vi "Run_Device.vi"(8 "error in (no error)":errorcluster, 10 "Message_command":T2, 11 "Command Queue":T3) -> (0 "error out":errorcluster, 2 "dup Message_command":T2, 3 "dup Command Queue":T3)   [LabVIEW 2020]
uses:
  Command_Queue.ctl
  Command_Message.ctl
  Device_List.ctl
panel:
  in  "Device":T1
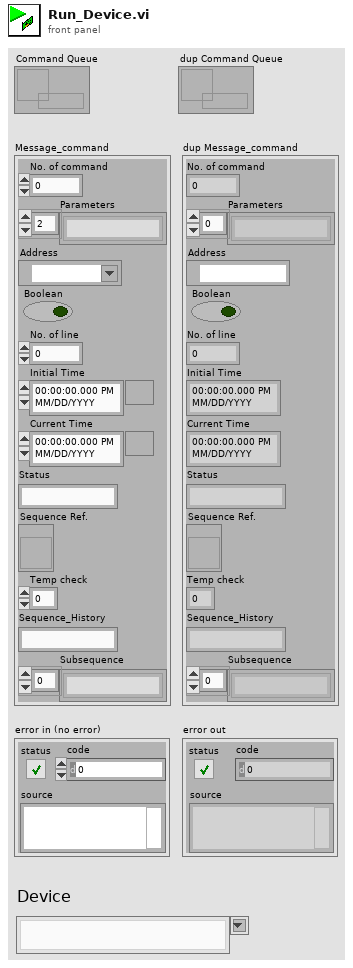
[diagram p1: front panel]
types:
  T1 = typedef "Device_List.ctl" = string
  T2 = typedef "Command_Message.ctl" = cluster{"No. of command":i32, "Parameters":string[], "Address":refnum<visa-resource-name>, "Boolean":bool, "No. of line":i32, "Initial Time":timestamp, "Current Time":timestamp, "Status":string, "Sequence Ref.":refnum<vi>, "Temp check":i32, "Sequence_History":string, "Subsequence":string[]}
  T3 = typedef "Command_Queue.ctl" = refnum<queue>
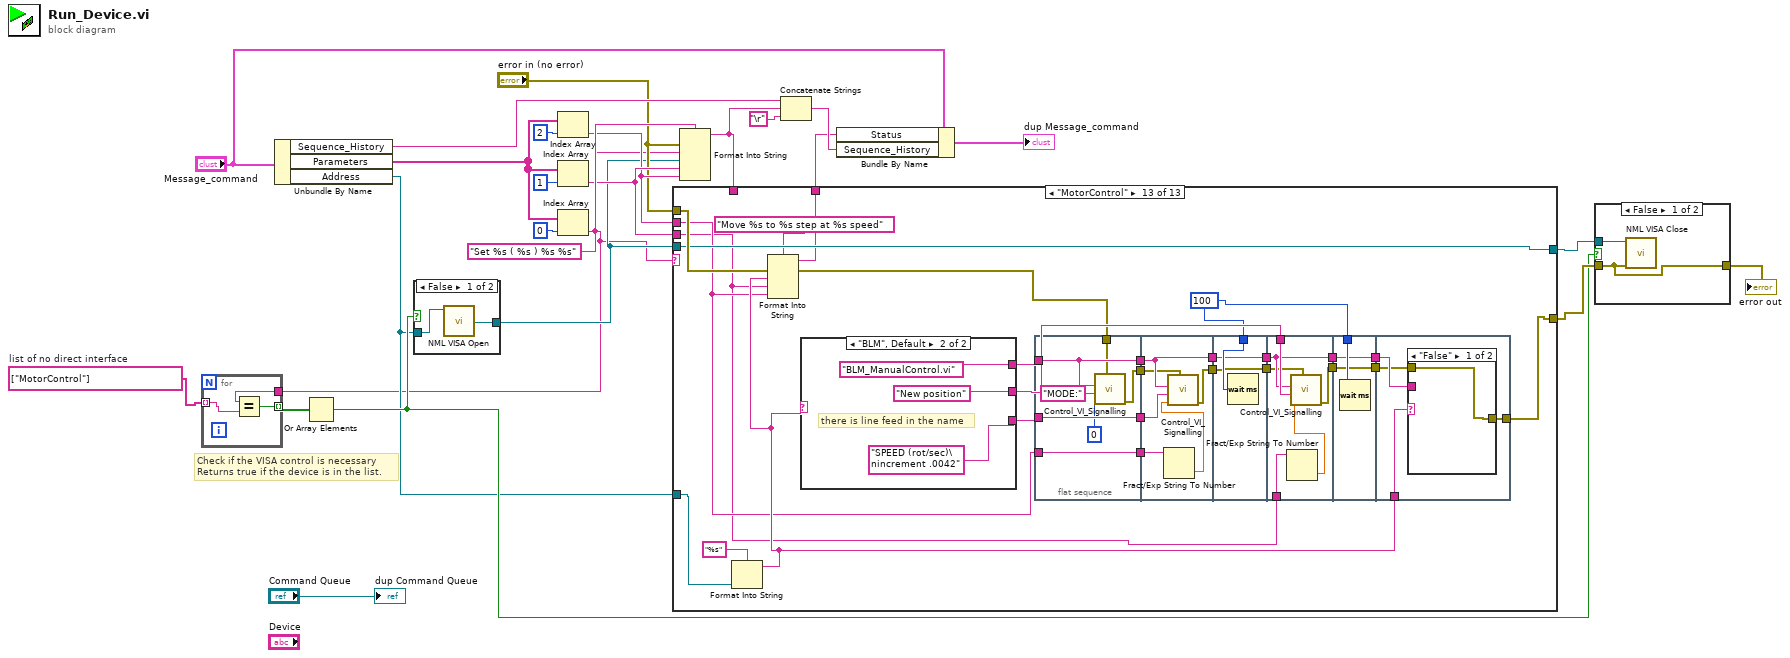
[diagram p0: block diagram]
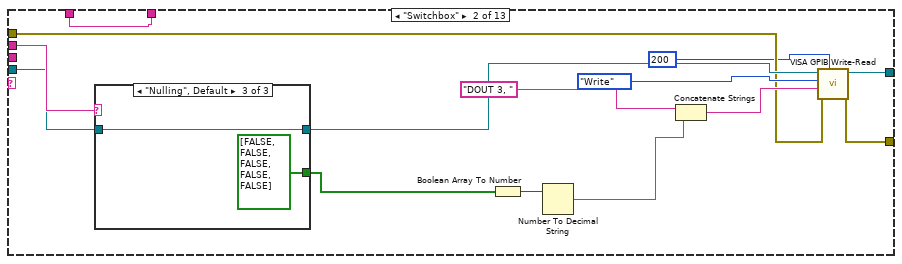
[diagram p5: hidden frame]
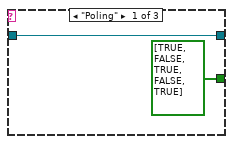
[diagram p6: hidden frame]
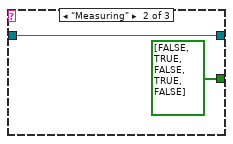
[diagram p7: hidden frame]
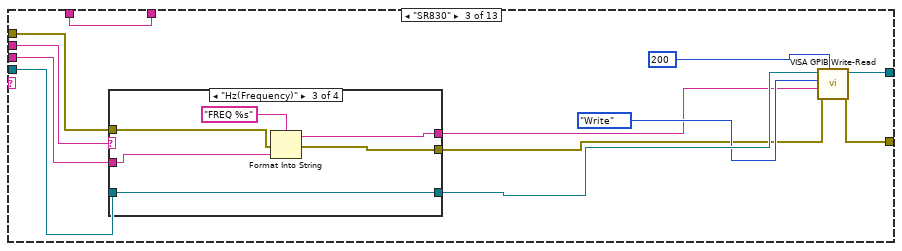
[diagram p8: hidden frame]
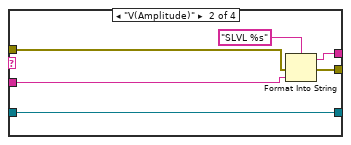
[diagram p10: hidden frame]
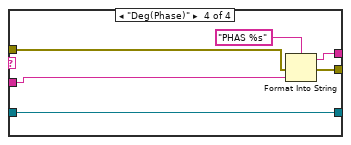
[diagram p11: hidden frame]
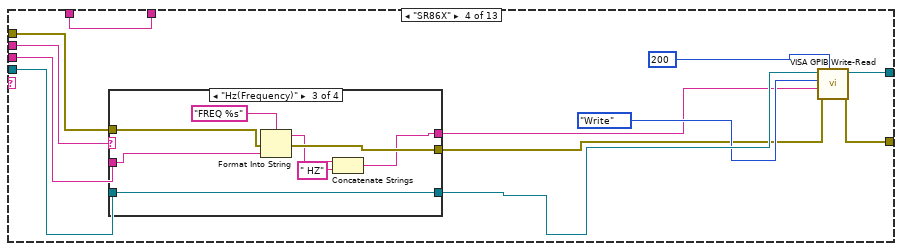
[diagram p12: hidden frame]
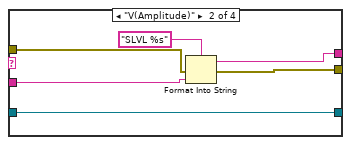
[diagram p14: hidden frame]
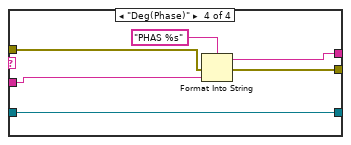
[diagram p15: hidden frame]
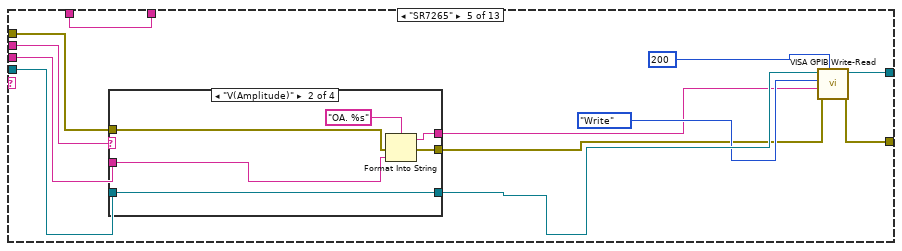
[diagram p16: hidden frame]
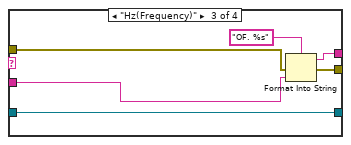
[diagram p18: hidden frame]
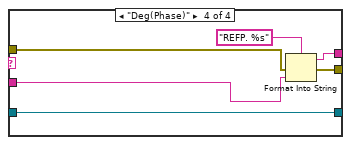
[diagram p19: hidden frame]
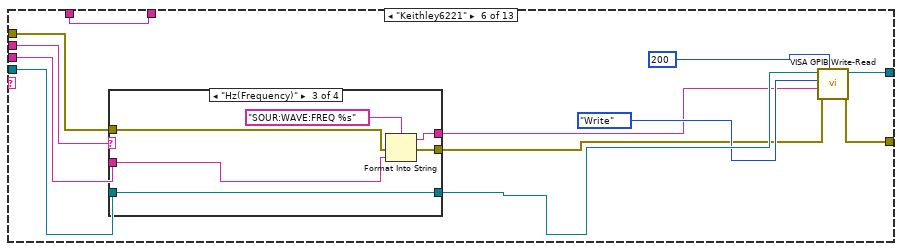
[diagram p20: hidden frame]
diagram:
  w7 = string[] ["MotorControl"]  # list of no direct interface
  # "Check if the VISA control is necessary\nReturns true if the device is in the list."
  n1 = Unbundle By Name("Message_command") -> ("Sequence_History"=w17:string, "Parameters"=w12:string[], "Address"=w4:refnum<visa-resource-name>)
  n2 = Index Array(array=w12, index=2) -> (element=w19:string)
  n3 = Index Array(array=w12, index=1) -> (element=w20:string)
  n4 = Index Array(array=w12, index=0) -> (element=w1:string)
  n5 = for {
    tunnel: w7 -> [w27] mode=indexing
    tunnel: w1 -> [w28]
    tunnel: [w26] -> w6 mode=indexing
    n6 = Equal?(x=w28, y=w27) -> (x = y?=w26:bool)
  }
  n7 = Or Array Elements(Boolean array=w6) -> (logical OR=w5:bool)
  n8 = case shown="False" w5 {
    tunnel: w4 -> [w30 w31]
    tunnel: [w29 w31] -> w11
    frame False {
      n9 = call "NML VISA Open.vi"("VISA resource name"=w30) -> ("VISA resource name out"=w29:refnum<visa-resource-name>)  [unwired: 9 in, 1 out]
    }
    frame True {
    }
  }
  n10 = Format Into String(format string="Set %s ( %s ) %s %s", error in="error in (no error)", w1, w11, w20, w19) -> (resulting string=w3:string)  [unwired: 1 in, 1 out]
  n11 = case shown="\"MotorControl\"" w1 {
    tunnel: w19 -> [_ w48 w66 w99 w134 w167 w202 w224 w315 w377 w440 w479 w521]
    tunnel: w20 -> [_ _ w64 w97 w132 w165 w200 w222 w313 w375 w436 w475 w520]
    tunnel: w11 -> [w33 w47 w63 w96 w131 w164 w199 w221 w312 w374 w437 w476 w524]
    tunnel: "error in (no error)" -> [w34 w39 w65 w98 w133 w166 w201 w223 w314 w376 w439 w478 w525]
    tunnel: [w34 w38 w58 w91 w126 w159 w194 w216 w307 w369 w438 w477 w512] -> w9
    tunnel: [w33 w36 w56 w89 w124 w157 w192 w214 w305 w367 w435 w474 w524] -> w10
    tunnel: w4 -> [_ _ _ _ _ _ _ _ _ _ _ _ w526]
    tunnel: w3 -> [w32 w35 w55 w88 w123 w156 w191 w213 w304 w366 w434 w473 _]
    tunnel: [w32 w35 w55 w88 w123 w156 w191 w213 w304 w366 w434 w473 w519] -> w2
    frame "False", Default {
    }
    frame "Switchbox" {
      n12 = case shown="\"Nulling\", Default" w48 {
        tunnel: w47 -> [w50 w51 w53]
        tunnel: [w50 w51 w53] -> w46
        tunnel: [bool[] [TRUE, FALSE, TRUE, FALSE, TRUE] bool[] [FALSE, TRUE, FALSE, TRUE, FALSE] bool[] [FALSE, FALSE, FALSE, FALSE, FALSE]] -> w41
        frame "Poling" {
        }
        frame "Measuring" {
        }
        frame "Nulling", Default {
        }
      }
      n13 = Boolean Array To Number(Boolean array=w41) -> (number=w42:u32)
      n14 = Number To Decimal String(number=w42) -> (decimal integer string=w44:string)  [unwired: 1 in]
      n15 = Concatenate Strings("DOUT 3, " ("string"), w44) -> (w40:string)
      n16 = call "VISA GPIB Write-Read.vi"("Wait (ms)"=u32 200 ("wait (mS)"), "error in (no error)"=w39, "Command"=w40, "Action"=enum16{"Write", "Read", "Write & Read"}."Write", "VISA resource name"=w46) -> ("error out"=w38:errorcluster, "dup VISA Session"=w36:refnum<visa-resource-name>)  [unwired: 3 in, 2 out]
    }
    frame "SR830" {
      n17 = case shown="\"Hz(Frequency)\"" w66 {
        selector: w66 -> [w67 _ _ _]
        tunnel: w65 -> [w69 w74 w80 w86]
        tunnel: [w69 w72 w78 w84] -> w59
        tunnel: w64 -> [_ w70 w76 w82]
        tunnel: [w67 w73 w79 w85] -> w60
        tunnel: w63 -> [w68 w71 w77 w83]
        tunnel: [w68 w71 w77 w83] -> w62
        frame Default {
        }
        frame "V(Amplitude)" {
          n18 = Format Into String(format string="SLVL %s", error in=w74, w70) -> (resulting string=w73:string, error out=w72:errorcluster)  [unwired: 1 in]
        }
        frame "Hz(Frequency)" {
          n19 = Format Into String(format string="FREQ %s", error in=w80, w76) -> (resulting string=w79:string, error out=w78:errorcluster)  [unwired: 1 in]
        }
        frame "Deg(Phase)" {
          n20 = Format Into String(format string="PHAS %s", error in=w86, w82) -> (resulting string=w85:string, error out=w84:errorcluster)  [unwired: 1 in]
        }
      }
      n21 = call "VISA GPIB Write-Read.vi"("Wait (ms)"=u32 200 ("wait (mS)"), "error in (no error)"=w59, "Command"=w60, "Action"=enum16{"Write", "Read", "Write & Read"}."Write", "VISA resource name"=w62) -> ("error out"=w58:errorcluster, "dup VISA Session"=w56:refnum<visa-resource-name>)  [unwired: 3 in, 2 out]
    }
    frame "SR86X" {
      n22 = case shown="\"Hz(Frequency)\"" w99 {
        selector: w99 -> [w100 _ _ _]
        tunnel: w98 -> [w102 w107 w115 w121]
        tunnel: [w102 w105 w114 w119] -> w92
        tunnel: w97 -> [_ w103 w112 w117]
        tunnel: [w100 w106 w109 w120] -> w93
        tunnel: w96 -> [w101 w104 w113 w118]
        tunnel: [w101 w104 w113 w118] -> w95
        frame Default {
        }
        frame "V(Amplitude)" {
          n23 = Format Into String(format string="SLVL %s", error in=w107, w103) -> (resulting string=w106:string, error out=w105:errorcluster)  [unwired: 1 in]
        }
        frame "Hz(Frequency)" {
          n24 = Format Into String(format string="FREQ %s", error in=w115, w112) -> (resulting string=w111:string, error out=w114:errorcluster)  [unwired: 1 in]
          n25 = Concatenate Strings(w111, " HZ" ("string")) -> (w109:string)
        }
        frame "Deg(Phase)" {
          n26 = Format Into String(format string="PHAS %s", error in=w121, w117) -> (resulting string=w120:string, error out=w119:errorcluster)  [unwired: 1 in]
        }
      }
      n27 = call "VISA GPIB Write-Read.vi"("Wait (ms)"=u32 200 ("wait (mS)"), "error in (no error)"=w92, "Command"=w93, "Action"=enum16{"Write", "Read", "Write & Read"}."Write", "VISA resource name"=w95) -> ("error out"=w91:errorcluster, "dup VISA Session"=w89:refnum<visa-resource-name>)  [unwired: 3 in, 2 out]
    }
    frame "SR7265" {
      n28 = case shown="\"V(Amplitude)\"" w134 {
        selector: w134 -> [w135 _ _ _]
        tunnel: w133 -> [w137 w142 w148 w154]
        tunnel: [w137 w140 w146 w152] -> w127
        tunnel: w132 -> [_ w138 w144 w150]
        tunnel: [w135 w141 w147 w153] -> w128
        tunnel: w131 -> [w136 w139 w145 w151]
        tunnel: [w136 w139 w145 w151] -> w130
        frame Default {
        }
        frame "V(Amplitude)" {
          n29 = Format Into String(format string="OA. %s", error in=w142, w138) -> (resulting string=w141:string, error out=w140:errorcluster)  [unwired: 1 in]
        }
        frame "Hz(Frequency)" {
          n30 = Format Into String(format string="OF. %s", error in=w148, w144) -> (resulting string=w147:string, error out=w146:errorcluster)  [unwired: 1 in]
        }
        frame "Deg(Phase)" {
          n31 = Format Into String(format string="REFP. %s", error in=w154, w150) -> (resulting string=w153:string, error out=w152:errorcluster)  [unwired: 1 in]
        }
      }
      n32 = call "VISA GPIB Write-Read.vi"("Wait (ms)"=u32 200 ("wait (mS)"), "error in (no error)"=w127, "Command"=w128, "Action"=enum16{"Write", "Read", "Write & Read"}."Write", "VISA resource name"=w130) -> ("error out"=w126:errorcluster, "dup VISA Session"=w124:refnum<visa-resource-name>)  [unwired: 3 in, 2 out]
    }
    frame "Keithley6221" {
      n33 = case shown="\"Hz(Frequency)\"" w167 {
        selector: w167 -> [w168 _ _ _]
        tunnel: w166 -> [w170 w174 w182 w187]
        tunnel: [w170 w172 w180 w185] -> w160
        tunnel: w165 -> [_ w176 w178 w189]
        tunnel: [w168 w173 w181 w186] -> w161
        tunnel: w164 -> [w169 w171 w179 w184]
        tunnel: [w169 w171 w179 w184] -> w163
        frame Default {
        }
        frame "mApp(ACCurrent)" {
          n34 = Fract/Exp String To Number(string=w176) -> (number=w175:dbl)  [unwired: 3 in, 1 out]
          n35 = Format Into String(format string="SOUR:WAVE:AMPL %fe-3", error in=w174, w175) -> (resulting string=w173:string, error out=w172:errorcluster)  [unwired: 1 in]
        }
        frame "Hz(Frequency)" {
          n36 = Format Into String(format string="SOUR:WAVE:FREQ %s", error in=w182, w178) -> (resulting string=w181:string, error out=w180:errorcluster)  [unwired: 1 in]
        }
        frame "mA(DCCurrent)" {
          n37 = Fract/Exp String To Number(string=w189) -> (number=w188:dbl)  [unwired: 3 in, 1 out]
          n38 = Format Into String(format string="CURR %fe-3", error in=w187, w188) -> (resulting string=w186:string, error out=w185:errorcluster)  [unwired: 1 in]
        }
      }
      n39 = call "VISA GPIB Write-Read.vi"("Wait (ms)"=u32 200 ("wait (mS)"), "error in (no error)"=w160, "Command"=w161, "Action"=enum16{"Write", "Read", "Write & Read"}."Write", "VISA resource name"=w163) -> ("error out"=w159:errorcluster, "dup VISA Session"=w157:refnum<visa-resource-name>)  [unwired: 3 in, 2 out]
    }
    frame "AH2700A" {
      n40 = case shown="\"Hz(Frequency)\"" w202 {
        selector: w202 -> [w203 _]
        tunnel: w201 -> [w205 w209]
        tunnel: [w205 w207] -> w195
        tunnel: w200 -> [_ w211]
        tunnel: [w203 w208] -> w196
        tunnel: w199 -> [w204 w206]
        tunnel: [w204 w206] -> w198
        frame Default {
        }
        frame "Hz(Frequency)" {
          n41 = Fract/Exp String To Number(string=w211) -> (number=w210:dbl)  [unwired: 3 in, 1 out]
          n42 = Format Into String(format string="FREQUENCY %f", error in=w209, w210) -> (resulting string=w208:string, error out=w207:errorcluster)  [unwired: 1 in]
        }
      }
      n43 = call "VISA GPIB Write-Read.vi"("Wait (ms)"=u32 200 ("wait (mS)"), "error in (no error)"=w195, "Command"=w196, "Action"=enum16{"Write", "Read", "Write & Read"}."Write", "VISA resource name"=w198) -> ("error out"=w194:errorcluster, "dup VISA Session"=w192:refnum<visa-resource-name>)  [unwired: 3 in, 2 out]
    }
    frame "LakeShore336" {
      n44 = case shown="\"loop1\"" w224 {
        selector: w224 -> [w225 _ _ _ _ _ _]
        tunnel: w223 -> [w227 w228 w238 w252 w266 w280 w294]
        tunnel: [w227 w228 w238 w252 w266 w280 w294] -> w217
        tunnel: w222 -> [_ w232 w242 w255 w269 w283 w297]
        tunnel: [w225 w229 w239 w253 w267 w281 w295] -> w218
        tunnel: w221 -> [w226 w233 w243 w256 w270 w284 w298]
        tunnel: [w226 w233 w243 w256 w270 w284 w298] -> w220
        frame Default {
        }
        frame "loop1" {
          n45 = case shown="\"high\", Default" w232 {
            tunnel: ["0" ("format string") "1" ("format string") "2" ("format string") "3" ("format string")] -> w230
            frame "off" {
            }
            frame "low" {
            }
            frame "med" {
            }
            frame "high", Default {
            }
          }
          n46 = Concatenate Strings("RANGE 1," ("format string"), w230) -> (w229:string)
        }
        frame "loop2" {
          n47 = case shown="\"high\", Default" w242 {
            tunnel: ["0" ("format string") "1" ("format string") "2" ("format string") "3" ("format string")] -> w240
            frame "off" {
            }
            frame "low" {
            }
            frame "med" {
            }
            frame "high", Default {
            }
          }
          n48 = Concatenate Strings("RANGE 2," ("format string"), w240) -> (w239:string)
        }
        frame "Asensor" {
          n49 = case shown="\"100kohm\"" w255 {
            tunnel: ["1, 8, " ("string") "0, 8, " ("string") "0, 7, " ("string") "0, 6, " ("string") "0, 5, " ("string")] -> w249
            frame "auto", Default {
            }
            frame "100kohm" {
            }
            frame "30kohm" {
            }
            frame "10kohm" {
            }
            frame "3kohm" {
            }
          }
          n50 = Concatenate Strings("INTYPE " ("format string"), "A " ("string"), "3, " ("string"), w249, "1, 1" ("string")) -> (w253:string)
        }
        frame "Bsensor" {
          n51 = case shown="\"100kohm\"" w269 {
            tunnel: ["1, 8, " ("string") "0, 8, " ("string") "0, 7, " ("string") "0, 6, " ("string") "0, 5, " ("string")] -> w263
            frame "auto", Default {
            }
            frame "100kohm" {
            }
            frame "30kohm" {
            }
            frame "10kohm" {
            }
            frame "3kohm" {
            }
          }
          n52 = Concatenate Strings("INTYPE " ("format string"), "B " ("string"), "3, " ("string"), w263, "1, 1" ("string")) -> (w267:string)
        }
        frame "Csensor" {
          n53 = case shown="\"100kohm\"" w283 {
            tunnel: ["1, 8, " ("string") "0, 8, " ("string") "0, 7, " ("string") "0, 6, " ("string") "0, 5, " ("string")] -> w277
            frame "auto", Default {
            }
            frame "100kohm" {
            }
            frame "30kohm" {
            }
            frame "10kohm" {
            }
            frame "3kohm" {
            }
          }
          n54 = Concatenate Strings("INTYPE " ("format string"), "C " ("string"), "3, " ("string"), w277, "1, 1" ("string")) -> (w281:string)
        }
        frame "Dsensor" {
          n55 = case shown="\"100kohm\"" w297 {
            tunnel: ["1, 8, " ("string") "0, 8, " ("string") "0, 7, " ("string") "0, 6, " ("string") "0, 5, " ("string")] -> w291
            frame "auto", Default {
            }
            frame "100kohm" {
            }
            frame "30kohm" {
            }
            frame "10kohm" {
            }
            frame "3kohm" {
            }
          }
          n56 = Concatenate Strings("INTYPE " ("format string"), "D " ("string"), "3, " ("string"), w291, "1, 1" ("string")) -> (w295:string)
        }
      }
      n57 = call "VISA GPIB Write-Read.vi"("Wait (ms)"=u32 200 ("wait (mS)"), "error in (no error)"=w217, "Command"=w218, "Action"=enum16{"Write", "Read", "Write & Read"}."Write", "VISA resource name"=w220) -> ("error out"=w216:errorcluster, "dup VISA Session"=w214:refnum<visa-resource-name>)  [unwired: 3 in, 2 out]
    }
    frame "LakeShore370" {
      n58 = case shown="\"Hrange\"" w315 {
        selector: w315 -> [w316 _ _]
        tunnel: w314 -> [w318 w328 w359]
        tunnel: [w318 w328 w359] -> w308
        tunnel: w313 -> [_ w321 w356]
        tunnel: [w316 w329 w360] -> w309
        tunnel: w312 -> [w317 w331 w343]
        tunnel: [w317 w331 w343] -> w311
        frame Default {
        }
        frame "Hrange" {
          w325 = string[] ["off", "31.6uA", "100uA", "316uA", "1mA", "3.16mA", "10mA", "31.6mA", "100mA"]  # 370 heater
          n59 = Match Pattern(string=w321, regular expression="::") -> (after substring=w323:string)  [unwired: 1 in, 3 out]
          n60 = Match Pattern(string=w323, regular expression="Hrange") -> (before substring=w320:string)  [unwired: 1 in, 3 out]
          n61 = call <vilib>:"Trim Whitespace.vi"("string"=w320) -> ("trimmed string"=w319:string)  [unwired: 1 in]
          n62 = Search 1D Array(1D array=w325, element=w319) -> (index of element=w327:i32)  [unwired: 1 in]
          n63 = Number To Decimal String(number=w327) -> (decimal integer string=w326:string)  [unwired: 1 in]
          n64 = Concatenate Strings("HTRRNG " ("format string"), w326) -> (w329:string)
        }
        frame "ResCurrentRange" {
          w335 = "," ("string")
          w354 = "::" ("regular expression")
          w358 = string[] ["1pA", "3.16pA", "10pA", "31.6pA", "100pA", "316pA", "1nA", "3.16nA", "10nA", "31.6nA", "100nA", "316nA", "1uA", "3.16uA", "10uA", "31.6uA", "100uA", "316uA", "1mA", "3.16mA", "10mA", "31.6mA"]  # 370 current
          # "0: autorange"
          n65 = Match Pattern(string=w356, regular expression=w354) -> (before substring=w347:string, after substring=w355:string)  [unwired: 1 in, 2 out]
          n66 = Match Pattern(string=w355, regular expression=w354) -> (before substring=w350:string, after substring=w353:string)  [unwired: 1 in, 2 out]
          n67 = Match Pattern(string=w347, regular expression="_") -> (after substring=w345:string)  [unwired: 1 in, 3 out]
          n68 = call <vilib>:"Trim Whitespace.vi"("string"=w350) -> ("trimmed string"=w336:string)  [unwired: 1 in]
          n69 = Match Pattern(string=w353, regular expression="ResCurrentRange") -> (before substring=w351:string)  [unwired: 1 in, 3 out]
          n70 = call <vilib>:"Trim Whitespace.vi"("string"=w351) -> ("trimmed string"=w337:string)  [unwired: 1 in]
          n71 = Search 1D Array(1D array=w358, element=w336) -> (index of element=w357:i32)  [unwired: 1 in]
          n72 = Search 1D Array(1D array=string[] ["auto", "2milliohm", "6.32milliohm", "20milliohm", "63.2milliohm", "200milliohm", "632milliohm", "2ohm", "6.32ohm", "20ohm", "63.2ohm", "200ohm", "632ohm", "2kohm", "6.32kohm", "20kohm", "63.2kohm", "200kohm", "632kohm", "2megaohm", "6.32megaohm", "20megaohm", "63.2megaohm"] ("370 R"), element=w337) -> (index of element=w333:i32)  [unwired: 1 in]
          n73 = Equal To 0?(x=w333) -> (x = 0?=w332:bool)
          n74 = Increment(x=w357) -> (x+1=w348:i32)
          n75 = case shown="False" w332 {
            tunnel: w333 -> [w363 w365]
            tunnel: [w363 w365] -> w341
            tunnel: [0 ("index of element") 1 ("index of element")] -> w339
            frame False {
            }
            frame True {
            }
          }
          n76 = Number To Decimal String(number=w348) -> (decimal integer string=w342:string)  [unwired: 1 in]
          n77 = Number To Decimal String(number=w341) -> (decimal integer string=w340:string)  [unwired: 1 in]
          n78 = Number To Decimal String(number=w339) -> (decimal integer string=w338:string)  [unwired: 1 in]
          n79 = Concatenate Strings("RDGRNG " ("format string"), w345, w335, "1," ("string"), w342, w335, w340, w335, w338, w335, "0" ("string")) -> (w360:string)
        }
      }
      n80 = call "VISA GPIB Write-Read.vi"("Wait (ms)"=u32 200 ("wait (mS)"), "error in (no error)"=w308, "Command"=w309, "Action"=enum16{"Write", "Read", "Write & Read"}."Write", "VISA resource name"=w311) -> ("error out"=w307:errorcluster, "dup VISA Session"=w305:refnum<visa-resource-name>)  [unwired: 3 in, 2 out]
    }
    frame "LakeShore372" {
      n81 = case shown="\"ResCurrentRange\"" w377 {
        selector: w377 -> [w378 _ _]
        tunnel: w376 -> [w380 w390 w425]
        tunnel: [w380 w390 w425] -> w370
        tunnel: w375 -> [_ w383 w422]
        tunnel: [w378 w391 w426] -> w371
        tunnel: w374 -> [w379 w393 w413]
        tunnel: [w379 w393 w413] -> w373
        frame Default {
        }
        frame "Hrange" {
          w387 = string[] ["off", "31.6uA", "100uA", "316uA", "1mA", "3.16mA", "10mA", "31.6mA", "100mA"]  # 370 heater
          n82 = Match Pattern(string=w383, regular expression="::") -> (after substring=w385:string)  [unwired: 1 in, 3 out]
          n83 = Match Pattern(string=w385, regular expression="Hrange") -> (before substring=w382:string)  [unwired: 1 in, 3 out]
          n84 = call <vilib>:"Trim Whitespace.vi"("string"=w382) -> ("trimmed string"=w381:string)  [unwired: 1 in]
          n85 = Search 1D Array(1D array=w387, element=w381) -> (index of element=w389:i32)  [unwired: 1 in]
          n86 = Number To Decimal String(number=w389) -> (decimal integer string=w388:string)  [unwired: 1 in]
          n87 = Concatenate Strings("HTRRNG " ("format string"), w388) -> (w391:string)
        }
        frame "ResCurrentRange" {
          w395 = "," ("string")
          w419 = string[] ["auto", "2milliohm", "6.32milliohm", "20milliohm", "63.2milliohm", "200milliohm", "632milliohm", "2ohm", "6.32ohm", "20ohm", "63.2ohm", "200ohm", "632ohm", "2kohm", "6.32kohm", "20kohm", "63.2kohm", "200kohm", "632kohm", "2megaohm", "6.32megaohm", "20megaohm", "63.2megaohm"]  # 370 R
          w403 = "::" ("regular expression")
          w424 = string[] ["1pA", "3.16pA", "10pA", "31.6pA", "100pA", "316pA", "1nA", "3.16nA", "10nA", "31.6nA", "100nA", "316nA", "1uA", "3.16uA", "10uA", "31.6uA", "100uA", "316uA", "1mA", "3.16mA", "10mA", "31.6mA"]  # 370 current
          # "0: autorange"
          n88 = Match Pattern(string=w422, regular expression=w403) -> (before substring=w417:string, after substring=w404:string)  [unwired: 1 in, 2 out]
          n89 = Match Pattern(string=w404, regular expression=w403) -> (before substring=w402:string, after substring=w401:string)  [unwired: 1 in, 2 out]
          n90 = Match Pattern(string=w401, regular expression=w403) -> (before substring=w400:string, after substring=w421:string)  [unwired: 1 in, 2 out]
          n91 = Match Pattern(string=w417, regular expression="_") -> (after substring=w415:string)  [unwired: 1 in, 3 out]
          n92 = Match Pattern(string=w421, regular expression="ResCurrentRange") -> (before substring=w399:string)  [unwired: 1 in, 3 out]
          n93 = call <vilib>:"Trim Whitespace.vi"("string"=w402) -> ("trimmed string"=w408:string)  [unwired: 1 in]
          n94 = call <vilib>:"Trim Whitespace.vi"("string"=w399) -> ("trimmed string"=w398:string)  [unwired: 1 in]
          n95 = case shown="\"kelvin\", Default" w398 {
            tunnel: ["2" ("trimmed string") "1" ("trimmed string")] -> w394
            frame "ohm" {
            }
            frame "kelvin", Default {
            }
          }
          n96 = call <vilib>:"Trim Whitespace.vi"("string"=w400) -> ("trimmed string"=w409:string)  [unwired: 1 in]
          n97 = Search 1D Array(1D array=w424, element=w408) -> (index of element=w423:i32)  [unwired: 1 in]
          n98 = Search 1D Array(1D array=w419, element=w409) -> (index of element=w406:i32)  [unwired: 1 in]
          n99 = Equal To 0?(x=w406) -> (x = 0?=w405:bool)
          n100 = Increment(x=w423) -> (x+1=w418:i32)
          n101 = case shown="True" w405 {
            tunnel: w406 -> [w431 w433]
            tunnel: [w431 w433] -> w411
            tunnel: [0 ("index of element") 1 ("index of element")] -> w410
            frame False {
            }
            frame True {
            }
          }
          n102 = Number To Decimal String(number=w418) -> (decimal integer string=w412:string)  [unwired: 1 in]
          n103 = Number To Decimal String(number=w411) -> (decimal integer string=w396:string)  [unwired: 1 in]
          n104 = Number To Decimal String(number=w410) -> (decimal integer string=w397:string)  [unwired: 1 in]
          n105 = Concatenate Strings("INTYPE " ("format string"), w415, w395, "1," ("string"), w412, w395, w397, w395, w396, w395, "0" ("string"), w395, w394) -> (w426:string)
        }
      }
      n106 = call "VISA GPIB Write-Read.vi"("Wait (ms)"=u32 200 ("wait (mS)"), "error in (no error)"=w370, "Command"=w371, "Action"=enum16{"Write", "Read", "Write & Read"}."Write", "VISA resource name"=w373) -> ("error out"=w369:errorcluster, "dup VISA Session"=w367:refnum<visa-resource-name>)  [unwired: 3 in, 2 out]
    }
    frame "Keithley6517" {
      n107 = case shown="\"V(Amplitude)\"" w440 {
        tunnel: w439 -> [w452 w472]
        tunnel: [w443 w472] -> w438
        tunnel: w437 -> [w455 w471]
        tunnel: w436 -> [w451 _]
        tunnel: [w441 w471] -> w435
        frame "V(Amplitude)" {
          w447 = 10.0 ("y")
          n108 = call "VISA GPIB Write-Read.vi"("error in (no error)"=w452, "Command"="SOUR:Volt? " ("String to Write"), "Action"=enum16{"Write", "Read", "Write & Read"}."Write & Read", "VISA resource name"=w455) -> ("error out"=w444:errorcluster, "String Returned"=w450:string, "dup VISA Session"=w442:refnum<visa-resource-name>)  [unwired: 4 in, 1 out]
          n109 = Fract/Exp String To Number(string=w450) -> (number=w445:dbl)  [unwired: 3 in, 1 out]
          n110 = Fract/Exp String To Number(string=w451) -> (number=w449:dbl)  [unwired: 3 in, 1 out]
          n111 = Subtract(x=w449, y=w445) -> (x-y=w448:dbl)
          n112 = Divide(x=w448, y=w447) -> (x/y=w446:dbl)
          n113 = for {
            N: w447 -> [_]
            tunnel: w446 -> [w468]
            tunnel: w445 -> [w466]
            tunnel: w444 -> [w460]
            tunnel: [w458] -> w443
            shift-right: [w456] -> w441
            shift-left: w442 -> [w457]
            i -> [w470]
            n114 = Increment(x=w470) -> (x+1=w469:i32)
            n115 = Multiply(x=w468, y=w469) -> (x*y=w467:dbl)
            n116 = Add(x=w466, y=w467) -> (x+y=w465:dbl)
            n117 = Format Into String(format string="SOUR:Volt %f" ("String to Write"), error in=w460, w465) -> (resulting string=w459:string, error out=w461:errorcluster)  [unwired: 1 in]
            n118 = call "VISA GPIB Write-Read.vi"("Wait (ms)"=u32 200 ("wait (mS)"), "error in (no error)"=w461, "Command"=w459, "Action"=enum16{"Write", "Read", "Write & Read"}."Write", "VISA resource name"=w457) -> ("error out"=w458:errorcluster, "dup VISA Session"=w456:refnum<visa-resource-name>)  [unwired: 3 in, 2 out]
          }
        }
        frame Default {
        }
      }
    }
    frame "Keithley24XX" {
      n119 = case shown="\"V(Amplitude)\"" w479 {
        tunnel: w478 -> [w491 w511]
        tunnel: [w482 w511] -> w477
        tunnel: w476 -> [w494 w510]
        tunnel: w475 -> [w490 _]
        tunnel: [w480 w510] -> w474
        frame "V(Amplitude)" {
          w486 = 10.0 ("y")
          n120 = call "VISA GPIB Write-Read.vi"("error in (no error)"=w491, "Command"="SOUR1:Volt? " ("String to Write"), "Action"=enum16{"Write", "Read", "Write & Read"}."Write & Read", "VISA resource name"=w494) -> ("error out"=w483:errorcluster, "String Returned"=w489:string, "dup VISA Session"=w481:refnum<visa-resource-name>)  [unwired: 4 in, 1 out]
          n121 = Fract/Exp String To Number(string=w489) -> (number=w484:dbl)  [unwired: 3 in, 1 out]
          n122 = Fract/Exp String To Number(string=w490) -> (number=w488:dbl)  [unwired: 3 in, 1 out]
          n123 = Subtract(x=w488, y=w484) -> (x-y=w487:dbl)
          n124 = Divide(x=w487, y=w486) -> (x/y=w485:dbl)
          n125 = for {
            N: w486 -> [_]
            tunnel: w485 -> [w507]
            tunnel: w484 -> [w505]
            tunnel: w483 -> [w499]
            tunnel: [w497] -> w482
            shift-right: [w495] -> w480
            shift-left: w481 -> [w496]
            i -> [w509]
            n126 = Increment(x=w509) -> (x+1=w508:i32)
            n127 = Multiply(x=w507, y=w508) -> (x*y=w506:dbl)
            n128 = Add(x=w505, y=w506) -> (x+y=w504:dbl)
            n129 = Format Into String(format string="SOUR1:Volt %f" ("String to Write"), error in=w499, w504) -> (resulting string=w498:string, error out=w500:errorcluster)  [unwired: 1 in]
            n130 = call "VISA GPIB Write-Read.vi"("Wait (ms)"=u32 200 ("wait (mS)"), "error in (no error)"=w500, "Command"=w498, "Action"=enum16{"Write", "Read", "Write & Read"}."Write", "VISA resource name"=w496) -> ("error out"=w497:errorcluster, "dup VISA Session"=w495:refnum<visa-resource-name>)  [unwired: 3 in, 2 out]
          }
        }
        frame Default {
        }
      }
    }
    frame "MotorControl" {
      w533 = u32 100 ("milliseconds to wait")
      n131 = Format Into String(format string="%s", w526) -> (resulting string=w522:string)  [unwired: 2 in, 1 out]
      n132 = Format Into String(format string="Move %s to %s step at %s speed", error in=w525, w522, w520, w521) -> (resulting string=w519:string, error out=w518:errorcluster)  [unwired: 1 in]
      n133 = case shown="\"BLM\", Default" w522 {
        tunnel: ["Stepper Mover.vi" ("Target VI name") "BLM_ManualControl.vi" ("Target VI name")] -> w538
        tunnel: ["Velocity" ("Target VI name") "SPEED (rot/sec)\nincrement .0042" ("Target VI name")] -> w537
        tunnel: ["Move to  Top Position (deg)" ("Target VI name") "New position" ("Target VI name")] -> w534
        frame "IMS" {
          (unwired) "Current Top Position" ("Target VI name")
        }
        frame "BLM", Default {
          # "there is line feed in the name"
        }
      }
      n134 = flat-sequence {
        tunnel: w521 -> [w550]
        tunnel: w537 -> [w551]
        tunnel: w538 -> [w549]
        tunnel: [w549] -> w530
        tunnel: [w551] -> w529
        tunnel: [w550] -> w528
        tunnel: w518 -> [w546]
        tunnel: [w545] -> w517
        tunnel: [w554] -> w536
        tunnel: w530 -> [w554]
        tunnel: w529 -> [w557]
        tunnel: w528 -> [w556]
        tunnel: w517 -> [w553]
        tunnel: [w552] -> w515
        tunnel: w533 -> [w560]
        tunnel: w536 -> [w559]
        tunnel: [w559] -> w535
        tunnel: [w558] -> w516
        tunnel: w515 -> [w558]
        tunnel: w535 -> [w563]
        tunnel: w534 -> [w566]
        tunnel: w520 -> [w565]
        tunnel: [w563] -> w532
        tunnel: w516 -> [w562]
        tunnel: [w561] -> w514
        tunnel: w533 -> [w569]
        tunnel: w532 -> [w568]
        tunnel: [w568] -> w531
        tunnel: w514 -> [w567]
        tunnel: [w567] -> w513
        tunnel: w531 -> [w573]
        tunnel: w522 -> [w572]
        tunnel: w513 -> [w571]
        tunnel: [w570] -> w512
        frame #0 {
          n135 = call "Control_VI_Signalling.vi"("error in (no error)"=w546, "Input Value"=0 ("index"), "Control Name"="MODE:", "Target VI name"=w549) -> ("error out"=w545:errorcluster)  [unwired: 7 in]
        }
        frame #1 {
          n136 = Fract/Exp String To Number(string=w556) -> (number=w555:dbl)  [unwired: 3 in, 1 out]
          n137 = call "Control_VI_Signalling.vi"("error in (no error)"=w553, "Input Value"=w555, "Control Name"=w557, "Target VI name"=w554) -> ("error out"=w552:errorcluster)  [unwired: 7 in]
        }
        frame #2 {
          n138 = Wait (ms)(milliseconds to wait=w560) -> ()  [unwired: 1 out]
        }
        frame #3 {
          n139 = Fract/Exp String To Number(string=w565) -> (number=w564:dbl)  [unwired: 3 in, 1 out]
          n140 = call "Control_VI_Signalling.vi"("error in (no error)"=w562, "Input Value"=w564, "Control Name"=w566, "Target VI name"=w563) -> ("error out"=w561:errorcluster)  [unwired: 7 in]
        }
        frame #4 {
          n141 = Wait (ms)(milliseconds to wait=w569) -> ()  [unwired: 1 out]
        }
        frame #5 {
          n142 = case shown="\"False\"" w572 {
            tunnel: w573 -> [_ w579]
            tunnel: w571 -> [w574 w576]
            tunnel: [w574 w575] -> w570
            frame "False" {
            }
            frame "BLM", Default {
              n143 = call "Control_VI_Signalling.vi"("error in (no error)"=w576, "Input Value"=TRUE, "Control Name"="Run" ("Target VI name"), "Target VI name"=w579) -> ("error out"=w575:errorcluster)  [unwired: 7 in]
            }
          }
        }
      }
    }
  }
  n144 = Concatenate Strings(w17, w3, "\r") -> (w15:string)
  n145 = Bundle By Name(cluster="Message_command", "Status"=w2, "Sequence_History"=w15) -> (→"dup Message_command":T2)
  n146 = case shown="False" w5 {
    tunnel: w10 -> [w581 _]
    tunnel: w9 -> [w580 w582]
    tunnel: [w580 w582] -> w8
    frame False {
      n147 = call "NML VISA Close.vi"("Error In"=w580, "VISA resource name"=w581) -> ()  [unwired: 9 in, 1 out]
    }
    frame True {
    }
  }
  "error out" <- w8
  "dup Command Queue" <- "Command Queue"
